vi "Save_Destinations_Core.vi"(8 "error in (no error)":errorcluster, 10 "commonPath":path, 11 "AB_Build in":refnum<class "AB_Build.lvclass">) -> (0 "error out":errorcluster, 3 "AB_Build out":refnum<class "AB_Build.lvclass">)   [LabVIEW 2020, in "AB_Build.lvclass"]
uses:
  <vilib>/AppBuilder/AB_Classes/Build/AB_Build.lvclass
  <vilib>/AppBuilder/AB_Classes/Build/AB_Build.lvclass/AB_Build.ctl
  <vilib>/AppBuilder/AB_Classes/Destination/AB_Destination.lvclass
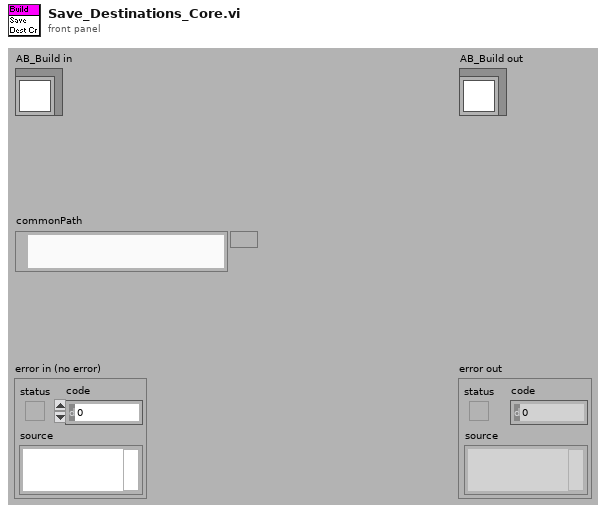
[diagram p1: front panel]
types:
  T1 = typedef "ItemRef.ctl" = u64
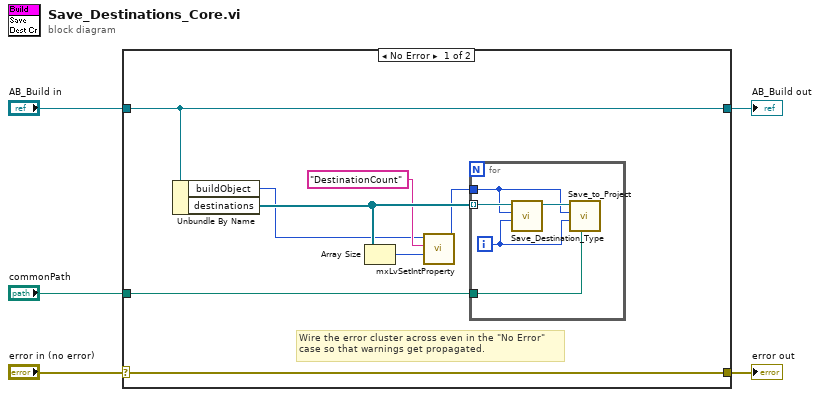
[diagram p0: block diagram]
diagram:
  n1 = case shown="No Error" "error in (no error)" {
    selector: "error in (no error)" -> [w13 w20]
    tunnel: [w13 w20] -> w4
    tunnel: [w8 w19] -> w2
    tunnel: "AB_Build in" -> [w8 w19]
    tunnel: "commonPath" -> [w7 _]
    frame No Error {
      # "Wire the error cluster across even in the \"No Error\"\ncase so that warnings get propagated."
      n2 = Unbundle By Name(w8) -> ("buildObject"=w6:T1, "destinations"=w11:refnum<class "AB_Destination.lvclass">[])
      n3 = Array Size(array=w11) -> (size(s)=w12:i32)
      n4 = call <resource>:"mxLvSetIntProperty.vi"("Value (0)"=w12, "Tag"="DestinationCount", "Item"=w6) -> ("Item"=w10:T1)  [unwired: 7 in, 1 out]
      n5 = for {
        tunnel: w11 -> [w18] mode=indexing
        tunnel: w10 -> [w16]
        tunnel: w7 -> [w14]
        i -> [w15]
        n6 = call-dynamic "Save_Destination_Type.vi"("index"=w15, "buildObject"=w16, "AB_Destination in"=w18) -> ("AB_Destination out"=w17:refnum<class "AB_Destination.lvclass">)  [unwired: 7 in, 1 out]
        n7 = call-dynamic "Save_to_Project.vi"("commonPath"=w14, "index"=w15, "buildObject"=w16, "AB_Destination in"=w17) -> ()  [unwired: 6 in, 2 out]
      }
    }
    frame Error {
    }
  }
  "error out" <- w4
  "AB_Build out" <- w2
